vi "Pockels Cal-AutoMeasure issue detector.vi"(9 "New Value (mW)":dbl, 11 "Pockels control voltage index":i32) -> (2 "Aborted by the user on detected issue":bool)   [LabVIEW 2020]
panel:
  out "appended array":dbl[](array[numeric])
  out "3 consecutive measurements are within +/-3mW of their previous one":bool
  out "3 consecutive measurements are within +/-2mW":bool
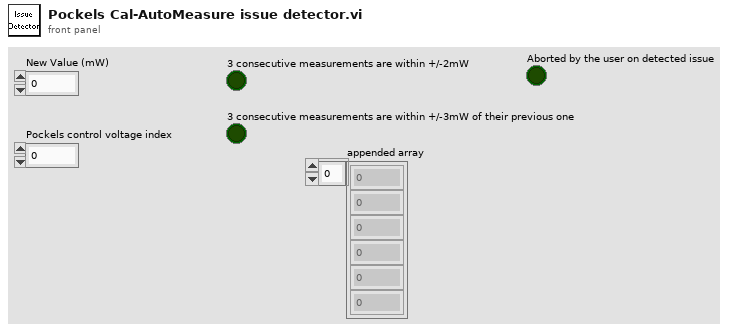
[diagram p1: front panel]
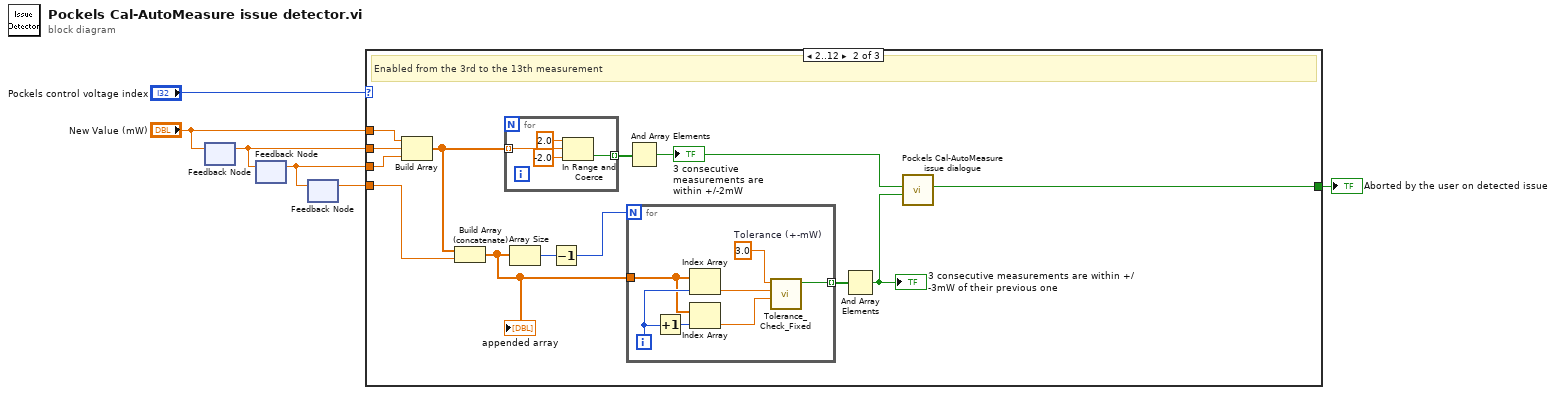
[diagram p0: block diagram]
diagram:
  n1 = feedback #1() -> (w4:dbl)  [unwired: 1 in]
  n2 = feedback-in #1("New Value (mW)") -> ()
  n3 = feedback #2() -> (w3:dbl)  [unwired: 1 in]
  n4 = feedback-in #2(w4) -> ()
  n5 = feedback #3() -> (w2:dbl)  [unwired: 1 in]
  n6 = feedback-in #3(w3) -> ()
  n7 = case shown="2..12" "Pockels control voltage index" {
    tunnel: "New Value (mW)" -> [_ w19 _]
    tunnel: w4 -> [_ w18 _]
    tunnel: w3 -> [_ w17 _]
    tunnel: w2 -> [_ w14 _]
    tunnel: [_ w7 _] -> w1
    frame 0, 1 {
      # "Disabled during the first and second measurement"
    }
    frame 2..12 {
      # "Enabled from the 3rd to the 13th measurement"
      n8 = Build Array(w19, w18, w17) -> (w15:dbl[])
      n9 = Build Array (concatenate)(w15, w14) -> (w13:dbl[])
      "appended array" <- w13
      n10 = for {
        tunnel: w15 -> [w28] mode=indexing
        tunnel: [w27] -> w16 mode=indexing
        n11 = In Range and Coerce(upper limit=2.0, x=w28, lower limit=-2.0) -> (In Range?=w27:bool)  [unwired: 1 out]
      }
      n12 = Array Size(array=w13) -> (size(s)=w12:i32)
      n13 = Decrement(x=w12) -> (x-1=w11:i32)
      n14 = for {
        N: w11 -> [_]
        tunnel: w13 -> [w23]
        tunnel: [w20] -> w10 mode=indexing
        i -> [w25]
        w21 = 3.0  # Tolerance (+-mW)
        n15 = Increment(x=w25) -> (x+1=w26:i32)
        n16 = Index Array(array=w23, index=w25) -> (element=w24:dbl)
        n17 = Index Array(array=w23, index=w26) -> (element=w22:dbl)
        n18 = call <userlib>:"Tolerance_Check_Fixed.vi"("Value to check"=w22, "Setpoint"=w24, "Tolerance (+-)"=w21) -> ("In Range"=w20:bool)  [unwired: 8 in]
      }
      n19 = And Array Elements(Boolean array=w16) -> (logical AND=w9:bool)
      "3 consecutive measurements are within +/-2mW" <- w9
      n20 = And Array Elements(Boolean array=w10) -> (logical AND=w8:bool)
      "3 consecutive measurements are within +/-3mW of their previous one" <- w8
      n21 = call "Pockels Cal-AutoMeasure issue dialogue.vi"("3 consecutive measurements are within +/-3mW of their previous one"=w8, "3 consecutive measurements are within +/-2mW"=w9) -> ("Aborted by the user on detected issue"=w7:bool)  [unwired: 9 in]
    }
    frame Default {
      # "Disabled for all measurements after the 13th one"
    }
  }
  "Aborted by the user on detected issue" <- w1
